vi "Main Action Que.vi"(7 "Action":enum16{"Initial", "Add", "Release"}(ring)=enum."Release", 8 "error in (no error)":errorcluster, 11 "Process":T1[](array[typedef])) -> (0 "error out":errorcluster, 3 "Process Que Out":refnum<queue>)   [LabVIEW 2019]
uses:
  Ctrl/Process Action Name.ctl
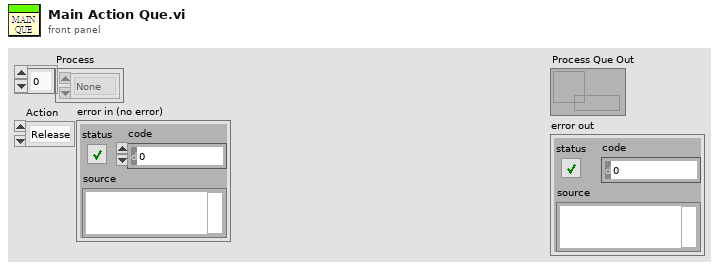
[diagram p1: front panel]
types:
  T1 = typedef "Process Action Name.ctl" = enum16{"None", "*******Initial*******", "*******Check Run*******", "*******Manual*******", "*******Others*******", "*******Exit*******", "Exit"}
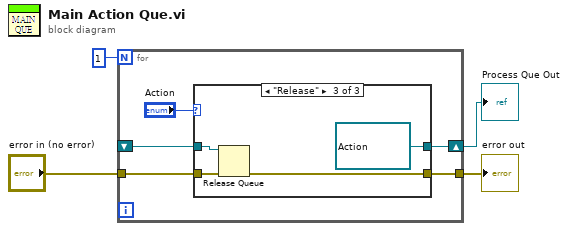
[diagram p0: block diagram]
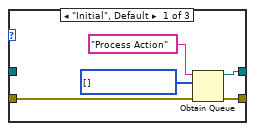
[diagram p2: hidden frame]
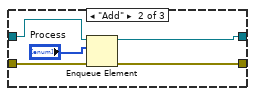
[diagram p3: hidden frame]
diagram:
  n1 = for {
    N: 1 -> [_]
    shift-right: [w9] -> w3
    shift-left: _ -> [w8]
    tunnel: "error in (no error)" -> [w6]
    tunnel: [w5] -> w1
    n2 = case shown="\"Release\"" "Action" {
      tunnel: [w12 w18 w22] -> w9
      tunnel: w8 -> [_ w19 w23]
      tunnel: w6 -> [w11 w15 w20]
      tunnel: [w10 w16 w21] -> w5
      frame "Initial", Default {
        w14 = T1[] [] items=["None", "*******Initial*******", "*******Check Run*******", "*******Manual*******", "*******Others*******", "*******Exit*******", "Exit"]
        n3 = Obtain Queue(name (unnamed)="Process Action", element data type=w14, error in (no error)=w11) -> (queue out=w12:refnum<queue>, error out=w10:errorcluster)  [unwired: 2 in, 1 out]
      }
      frame "Add" {
        n4 = Enqueue Element(queue=w19, element="Process", error in (no error)=w15) -> (queue out=w18:refnum<queue>, error out=w16:errorcluster)  [unwired: 1 in, 1 out]
      }
      frame "Release" {
        w22 = refnum<queue> refnum items=["None", "*******Initial*******", "*******Check Run*******", "*******Manual*******", "*******Others*******", "*******Exit*******", "Exit"] ("queue out")
        n5 = Release Queue(queue=w23, error in (no error)=w20) -> (error out=w21:errorcluster)  [unwired: 1 in, 2 out]
      }
    }
  }
  "Process Que Out" <- w3
  "error out" <- w1
